vi "name.get.vi"(11 "test-channel in":refnum<class "test-channel.lvclass">) -> (2 "name":string, 3 "test-channel out":refnum<class "test-channel.lvclass">)   [LabVIEW 2020, in "test-channel.lvclass"]
uses:
  test-channel.lvclass
  test-channel.lvclass/test-channel.ctl
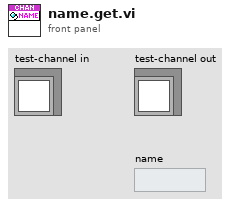
[diagram p1: front panel]
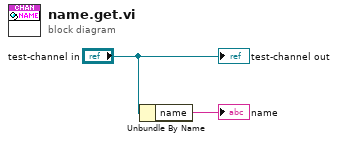
[diagram p0: block diagram]
diagram:
  n1 = Unbundle By Name("test-channel in") -> ("name"=→"name":string)
  "test-channel out" <- "test-channel in"
